vi "Flatten To String.vi"(8 "error in (no error)":errorcluster, 10 "Variant":variant, 11 "Serializer in":refnum<class "Serializer.lvclass">) -> (0 "error out":errorcluster, 2 "String":string, 3 "Serializer out":refnum<class "Serializer.lvclass">)   [LabVIEW 2019, in "JKI Serialization.lvlib" / "Serializer.lvclass"]
doc: "JKI Serialization 1.0.1.14\nTomi Maila - JKI\nCopyright (c) 2016, JKI"
uses:
  Serializer.lvclass
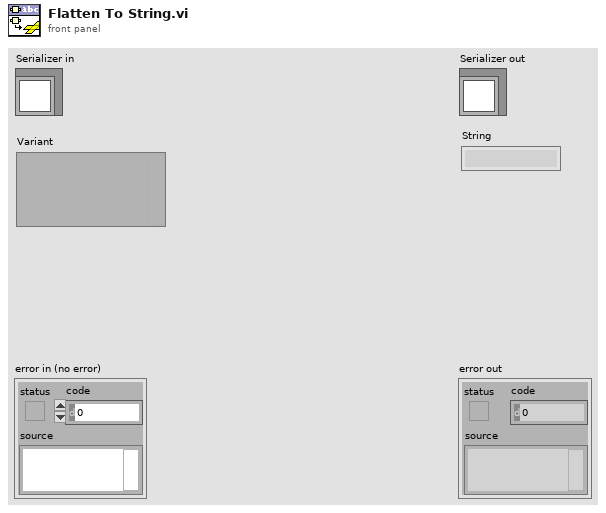
[diagram p1: front panel]
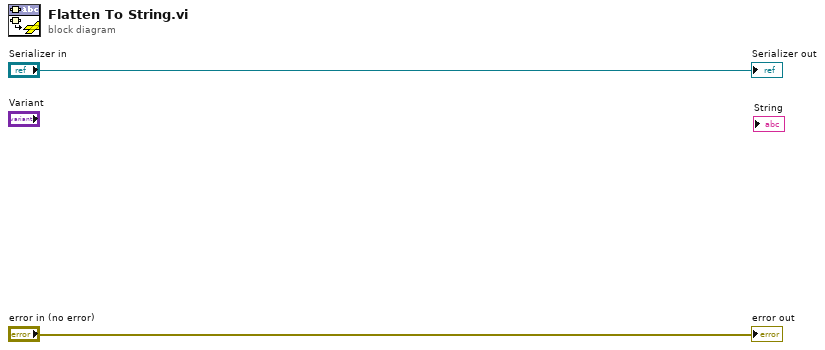
[diagram p0: block diagram]
diagram:
  "error out" <- "error in (no error)"
  "Serializer out" <- "Serializer in"
